vi "SRDG535.evt Call Set Delay.vi"(0 "i ref in":refnum<vi>, 2 "Generator Instance":string="N/A", 3 "Delay Settings":T1 {"CH D"."Delay (s)" format="%#_13g"; "CH D"."rel to" scale=0.0..3.0; "CH C"."Delay (s)" format="%#_13g"; "CH C"."rel to" scale=0.0..3.0; "CH B"."Delay (s)" format="%#_13g"; "CH B"."rel to" scale=0.0..3.0; "CH A"."Delay (s)" format="%#_13g"; "CH A"."rel to" scale=0.0..3.0}, 5 "error IO":errorcluster) -> (14 "i ref out":refnum<vi>, 19 "error out":errorcluster)   [LabVIEW 2014, in "SRDG535.lvlib"]
doc: "This VI sends a simple event call."
uses:
  SRDG535.lvlib
  SRDG535.Delay.ctl
  CS_Core/CSSystem/CoreLib/CoreLib.short 2 byte array.vi
  CS_Core/CSSystem/CoreLib/CoreLib.double 2 byte array.vi
  CS_Core/CSSystem/CoreLib/CoreLib.lvlib
  CS_Core/BaseProcess/BaseProcess.lvlib
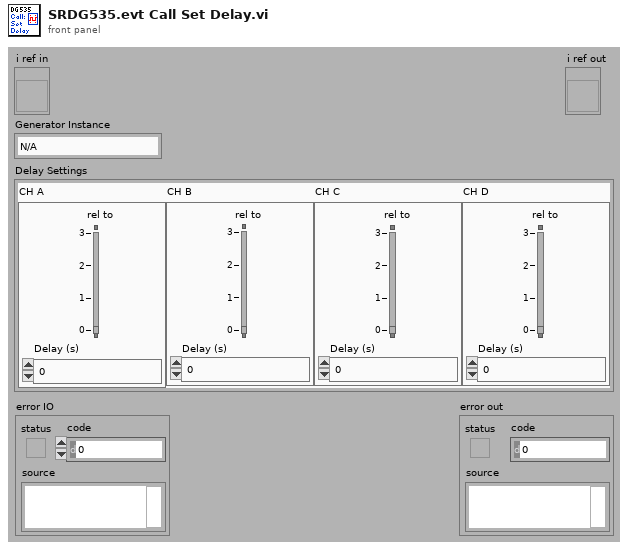
[diagram p1: front panel]
types:
  T1 = typedef "SRDG535.lvlib/SRDG535.Delay.ctl" = cluster{"CH A":cluster{"rel to":u32, "Delay (s)":dbl}, "CH B":cluster{"rel to":u32, "Delay (s)":dbl}, "CH C":cluster{"rel to":u32, "Delay (s)":dbl}, "CH D":cluster{"rel to":u32, "Delay (s)":dbl}}
  T2 = typedef "CoreDefs.rawDataType.ctl" = i8[]
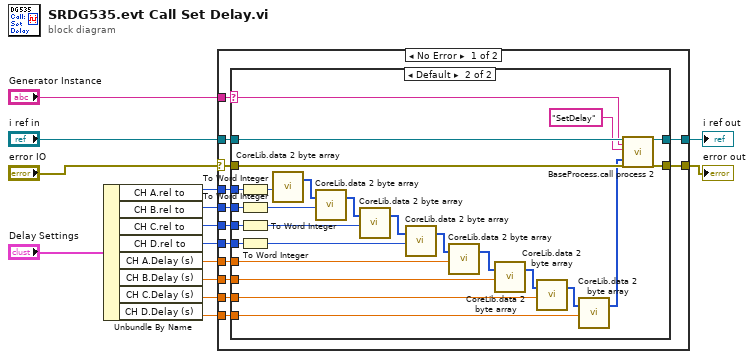
[diagram p0: block diagram]
diagram:
  n1 = Unbundle By Name("Delay Settings") -> ("CH A.rel to"=w8:u32, "CH B.rel to"=w7:u32, "CH C.rel to"=w6:u32, "CH D.rel to"=w5:u32, "CH A.Delay (s)"=w4:dbl, "CH B.Delay (s)"=w3:dbl, "CH C.Delay (s)"=w2:dbl, "CH D.Delay (s)"=w1:dbl)
  n2 = case shown="No Error" "error IO" {
    selector: "error IO" -> [w27 w56]
    tunnel: "Generator Instance" -> [w15 _]
    tunnel: [w26 w56] -> w14
    tunnel: [w24 w57] -> w13
    tunnel: w1 -> [w16 _]
    tunnel: w2 -> [w17 _]
    tunnel: w3 -> [w18 _]
    tunnel: w4 -> [w19 _]
    tunnel: w5 -> [w20 _]
    tunnel: w6 -> [w21 _]
    tunnel: w7 -> [w22 _]
    tunnel: w8 -> [w23 _]
    tunnel: "i ref in" -> [w25 w57]
    frame No Error {
      n3 = case shown="Default" w15 {
        selector: w15 -> [_ w30]
        tunnel: w27 -> [w28 w55]
        tunnel: [w28 w54] -> w26
        tunnel: w25 -> [w29 w53]
        tunnel: [w29 w52] -> w24
        tunnel: w23 -> [_ w44]
        tunnel: w22 -> [_ w43]
        tunnel: w21 -> [_ w42]
        tunnel: w20 -> [_ w41]
        tunnel: w19 -> [_ w35]
        tunnel: w18 -> [_ w34]
        tunnel: w17 -> [_ w33]
        tunnel: w16 -> [_ w32]
        frame "", "N/A" {
        }
        frame Default {
          n4 = To Word Integer(number=w44) -> (16bit integer=w40:i16)
          n5 = To Word Integer(number=w43) -> (16bit integer=w39:i16)
          n6 = To Word Integer(number=w42) -> (16bit integer=w38:i16)
          n7 = To Word Integer(number=w41) -> (16bit integer=w37:i16)
          n8 = call-poly "CoreLib.data 2 byte array.vi"("i16"=w40) -> ("byteArray out"=w47:T2)  [unwired: 18 in]
          n9 = call-poly "CoreLib.data 2 byte array.vi"("byteArray"=w47, "i16"=w39) -> ("byteArray out"=w46:T2)  [unwired: 17 in]
          n10 = call-poly "CoreLib.data 2 byte array.vi"("byteArray"=w46, "i16"=w38) -> ("byteArray out"=w45:T2)  [unwired: 17 in]
          n11 = call-poly "CoreLib.data 2 byte array.vi"("byteArray"=w45, "i16"=w37) -> ("byteArray out"=w36:T2)  [unwired: 17 in]
          n12 = call-poly "CoreLib.data 2 byte array.vi"("byteArray"=w36, "f64"=w35) -> ("byteArray out"=w50:T2)  [unwired: 17 in]
          n13 = call-poly "CoreLib.data 2 byte array.vi"("byteArray"=w50, "f64"=w34) -> ("byteArray out"=w49:T2)  [unwired: 17 in]
          n14 = call-poly "CoreLib.data 2 byte array.vi"("byteArray"=w49, "f64"=w33) -> ("byteArray out"=w48:T2)  [unwired: 17 in]
          n15 = call-poly "CoreLib.data 2 byte array.vi"("byteArray"=w48, "f64"=w32) -> ("byteArray out"=w31:T2)  [unwired: 17 in]
          n16 = call "BaseProcess.call process 2.vi"("i ref in"=w53, "Object"=w30, "Selector"="SetDelay", "Data"=w31, "error in (no error)"=w55) -> ("i ref out"=w52:refnum<vi>, "error out"=w54:errorcluster)  [unwired: 13 in]
        }
      }
    }
    frame Error {
    }
  }
  "error out" <- w14
  "i ref out" <- w13
